vi "dfd_CIC Comb Simu.vi"(5 "lag":i32, 7 "#stage":i32, 8 "history in":T1[](array[typedef]), 9 "Decimation?":bool, 10 "Bit to cut":i32[](array[numeric]), 11 "x":T1) -> (0 "history out":T1[](array[typedef]), 3 "y":T1)   [LabVIEW 2017, in "NI_DigFilter_FXP.lvlib"]
uses:
  <vilib>/addons/Digital Filter Design/NI_DigFilter_FXP.lvlib
  <vilib>/addons/Digital Filter Design/_Objects.llb/dfd_Integer I160.ctl
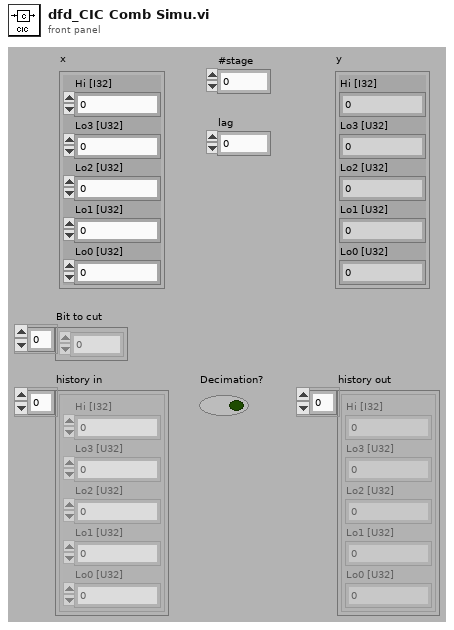
[diagram p1: front panel]
types:
  T1 = typedef "dfd_Integer I160.ctl" = cluster{"Hi [I32]":i32, "Lo3 [U32]":u32, "Lo2 [U32]":u32, "Lo1 [U32]":u32, "Lo0 [U32]":u32}
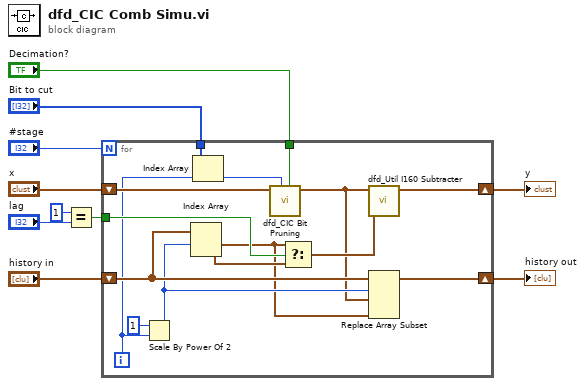
[diagram p0: block diagram]
diagram:
  n1 = Equal?(x=1, y="lag") -> (x = y?=w3:bool)
  n2 = for {
    N: "#stage" -> [_]
    shift-right: [w24] -> w6
    shift-left: "history in" -> [w23]
    shift-right: [w25] -> w9
    shift-left: "x" -> [w16]
    tunnel: w3 -> [w22]
    tunnel: "Decimation?" -> [w14]
    tunnel: "Bit to cut" -> [w12]
    i -> [w13]
    n3 = Scale By Power Of 2(n=1, x=w13) -> (x*2^n=w19:i32)
    n4 = Index Array(array=w23, index #1=w19) -> (element #1=w18:T1, element #2=w21:T1)  [unwired: 1 in]
    n5 = Index Array(array=w12, index=w13) -> (element=w11:i32)
    n6 = call <vilib>:"dfd_CIC Bit Pruning.vi"("cut?"=w14, "Bit to cut"=w11, "x"=w16) -> ("y"=w15:T1)  [unwired: 8 out]
    n7 = Select(t=w18, s=w22, f=w21) -> (s? t:f=w20:T1)
    n8 = call <vilib>:"dfd_Util I160 Subtracter.vi"("y [I160]"=w20, "x [I160]"=w15) -> ("x-y [I160]"=w25:T1)  [unwired: 9 out]
    n9 = Replace Array Subset(array=w23, new element #1=w15, index #1=w19, new element #2=w18) -> (w24:T1[])  [unwired: 1 in]
  }
  "y" <- w9
  "history out" <- w6
